vi "AD5781StepLogic.vi"(4 "invertDirection":bool, 6 "restart":bool, 8 "Start":i32 format="%032b", 9 "Step":i32 format="%032b") -> (2 "timedOut":bool)   [LabVIEW 2014]
uses:
  <vilib>/rvi/Emulation/niFpgaGetClockAttributes.vi
  <vilib>/rvi/Emulation/niFpgaSctlEmulationGetInTimedLoop.vi
  <vilib>/rvi/Emulation/niFpgaEmulationReportErrorSimple.vi
  Code/FPGA SPI_Globals.vi
  <vilib>/rvi/Emulation/niFpgaCriticalErrorInLSC.vi
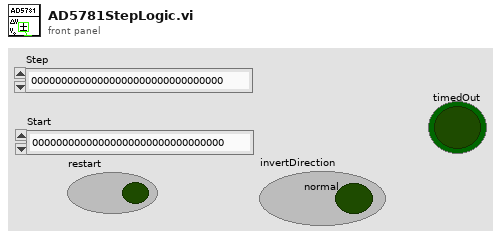
[diagram p1: front panel]
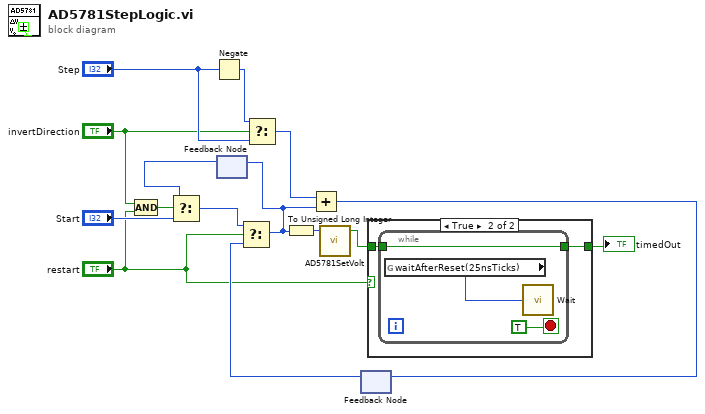
[diagram p0: block diagram]
diagram:
  n1 = Compound Arithmetic op=AND("invertDirection", "restart") -> (w2:bool)
  n2 = Negate(x="Step") -> (-x=w15:i32)
  n3 = feedback #1() -> (w1:i32)  [unwired: 1 in]
  n4 = Select(t=w1, s=w2, f="Start") -> (s? t:f=w5:i32)
  n5 = Select(t=w15, s="invertDirection", f="Step") -> (s? t:f=w13:i32)
  n6 = feedback #2() -> (w10:i32)  [unwired: 1 in]
  n7 = Select(t=w5, s="restart", f=w10) -> (s? t:f=w7:i32)
  n8 = feedback-in #1(w7) -> ()
  n9 = To Unsigned Long Integer(number=w7) -> (unsigned 32bit integer=w11:u32)
  n10 = Add(x=w13, y=w7) -> (x+y=w12:i32)
  n11 = call "AD5781SetVolt.vi"("SetVolt"=w11) -> ("timedOut"=w9:bool)  [unwired: 4 in]
  n12 = feedback-in #2(w12) -> ()
  n13 = case shown="True" "restart" {
    tunnel: w9 -> [w16 w18]
    tunnel: [w16 w17] -> w8
    frame False {
    }
    frame True {
      n14 = while {
        tunnel: w18 -> [w19]
        tunnel: [w19] -> w17
        stop <- TRUE stop-if-true
        n15 = global read "FPGA SPI_Globals.vi" "waitAfterReset(25nsTicks)"() -> (w21:u16)
        n16 = call "Wait"("Count(Ticks)"=w21) -> ()  [unwired: 1 out]
      }
    }
  }
  "timedOut" <- w8
